vi "Destroy Msg Event DVR.vi"(10 "Msg Event DVR":refnum<data-value>) -> (0 "error out":errorcluster)   [LabVIEW 2021, in "jettl.lvlib"]
uses:
  jettl.lvlib
  Actor/Msg/Msg.lvclass
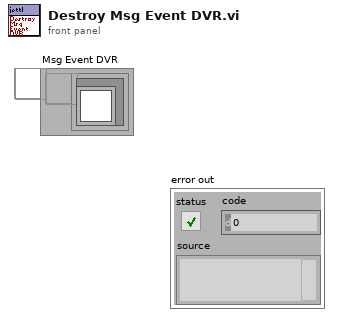
[diagram p1: front panel]
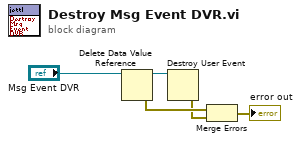
[diagram p0: block diagram]
diagram:
  n1 = Delete Data Value Reference(data value reference="Msg Event DVR") -> (data value=w2:refnum<user-event>, error out=w4:errorcluster)  [unwired: 1 in]
  n2 = Destroy User Event(user event=w2) -> (error out=w1:errorcluster)  [unwired: 1 in]
  n3 = Merge Errors(w4, w1) -> (→"error out":errorcluster)
